vi "_XNET Convert Time U64 1ns to LV.vi"(3 "Time U64 1ns":u64) -> (1 "Time LV":timestamp)   [LabVIEW 2018]
uses:
  nixlvapi.dll
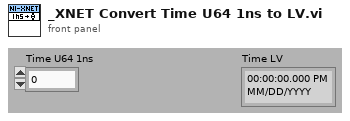
[diagram p1: front panel]
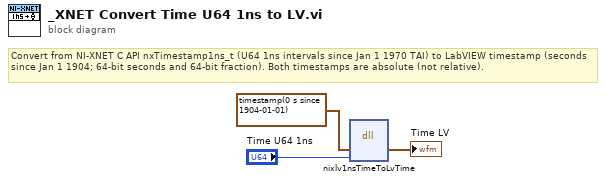
[diagram p0: block diagram]
diagram:
  # "Convert from NI-XNET C API nxTimestamp1ns_t (U64 1ns intervals since Jan 1 1970 TAI) to LabVIEW timestamp (seconds since Jan 1 1904; 64-bit seconds and 64-bit fraction). Both timestamps are absolute (not relative)."
  n1 = dll-call lib="nixlvapi.*" fn="nixlv1nsTimeToLvTime" label="Call Library"("lvTime"=timestamp(0 s since 1904-01-01) ("Time LV"), "cTime"="Time U64 1ns") -> ("lvTime"=→"Time LV":timestamp)  [unwired: 4 in, 3 out]
